vi "AR-Check-Gating.vi"(8 "error in":errorcluster, 10 "Zaber parameters":T3={"Device (dev axis)"="1 3", "Lockstep Group (1)"=1, "Units"=enum."millimeters", "Microstep Size"=4.21875, "Move (units)"=1500.0, "Direction(-1,1)"=0, "Speed (units/s)"=0.0}, 11 "Com ports":T2={"Zaber Com"="COM21", "MCU Com"="COM22", "Laser IP"=""}) -> (0 "error out":errorcluster, 1 "Timed Out":bool=TRUE, 2 "Time Delta (mS)":dbl, 3 "X Pos Triggered":dbl=1500.0)   [LabVIEW 2021]
uses:
  Automation/Zaber Stage/Controls/Zaber-parameters.ctl
  Controls/AR-Interlock-Data.ctl
  Controls/AR-Interlock-monitor-comands.ctl
  Controls/AR-axis-parameters.ctl
panel:
  out "Raw Output 3":string
  out "Raw Output 2":string
  out "Raw Output":string
  in  "Timeout (s)":u32=5
  out "Intlk Data Array":T1[](array[typedef])=[{"Application"="GI", "Msg#"=31, "uS time"=3584961232, "Gate"=FALSE, "Head"=FALSE, "Head Old"=FALSE, "Chamber Ena"=TRUE, "Profiler Ena"=FALSE, "OPower Ena"=FALSE, "Gate Ena"=TRUE, "Time Delta (mS)"=0.0, "Head F Edge"=FALSE}, {"Application"="GI", "Msg#"=32, "uS time"=3633481693, "Gate"=FALSE, "Head"=FALSE, "Head Old"=FALSE, "Chamber Ena"=TRUE, "Profiler Ena"=FALSE, "OPower Ena"=FALSE, "Gate Ena"=TRUE, "Time Delta (mS)"=48520.461, "Head F Edge"=FALSE}] {"Time Delta (mS)" format="%#_3g"}
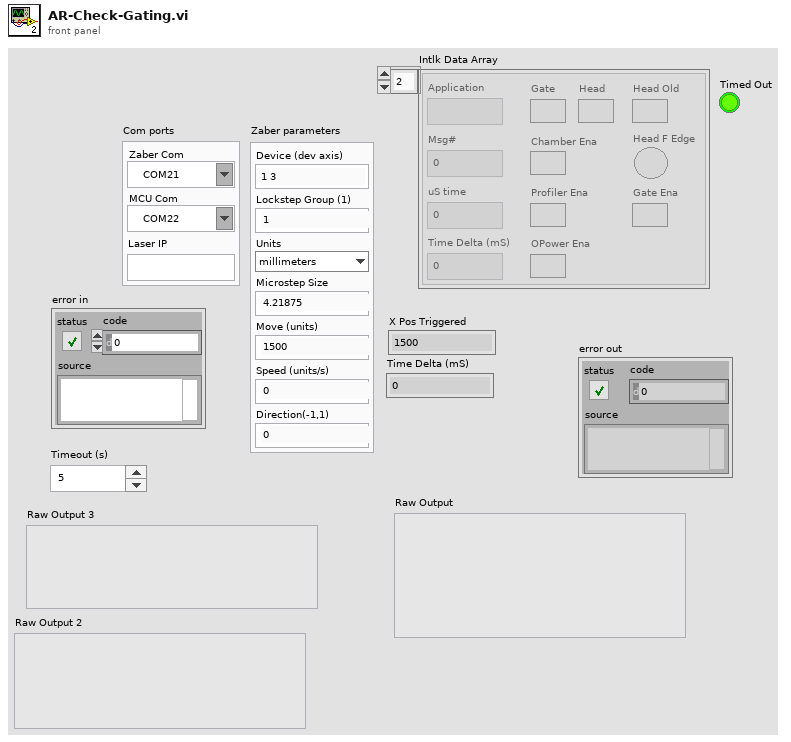
[diagram p1: front panel]
types:
  T1 = typedef "AR-Interlock-Data.ctl" = cluster{"Application":string, "Msg#":i32, "uS time":u32, "Gate":bool, "Head":bool, "Head Old":bool, "Chamber Ena":bool, "Profiler Ena":bool, "OPower Ena":bool, "Gate Ena":bool, "Time Delta (mS)":dbl, "Head F Edge":bool}
  T2 = cluster{"Zaber Com":refnum<visa-resource-name>, "MCU Com":refnum<visa-resource-name>, "Laser IP":string}
  T3 = typedef "Zaber-parameters.ctl" = cluster{"Device (dev axis)":string, "Lockstep Group (1)":u8, "Units":enum16{"microsteps", "microns", "millimeters", "inches", "degrees"}, "Microstep Size":dbl, "Move (units)":dbl, "Direction(-1,1)":i32, "Speed (units/s)":dbl}
  T4 = typedef "AR-Interlock-monitor-comands.ctl" = enum16{"Init", "Request", "Poll Serial", "Close", "Clear Data"}
  T5 = typedef "AR-axis-parameters.ctl" = cluster{"X":T3, "Y":T3}
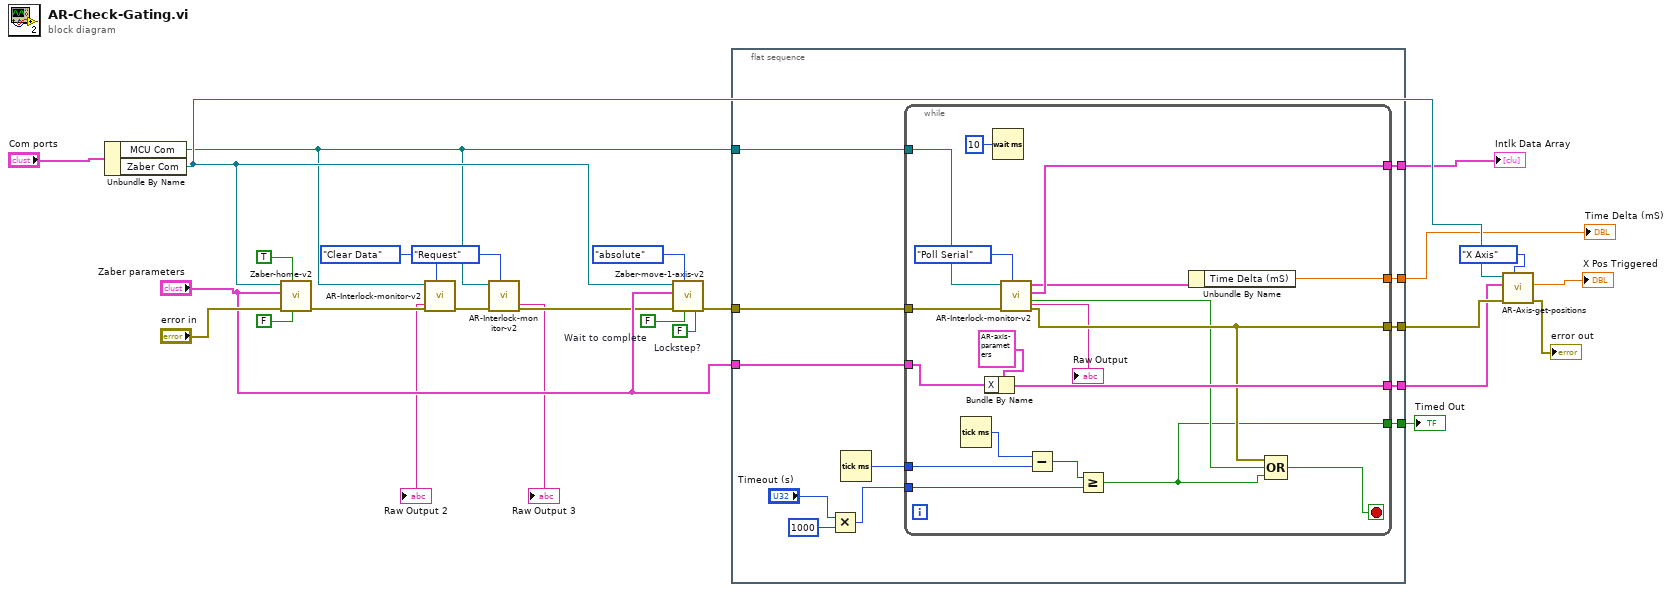
[diagram p0: block diagram]
diagram:
  w25 = FALSE  # Wait to complete
  w24 = FALSE  # Lockstep?
  n1 = Unbundle By Name("Com ports") -> ("MCU Com"=w5:refnum<visa-resource-name>, "Zaber Com"=w16:refnum<visa-resource-name>)
  n2 = call "Zaber-home-v2.vi"("Lockstep?"=FALSE, "Wait to complete"=TRUE, "error in"="error in", "Zaber parameters"="Zaber parameters", "Com Port"=w16) -> ("error out"=w19:errorcluster)  [unwired: 4 in, 2 out]
  n3 = call "AR-Interlock-monitor-v2.vi"("Action"=AR-Interlock-monitor-comands."Clear Data", "error in"=w19, "Inlk Com"=w5) -> ("error out"=w7:errorcluster, "Raw Output"=→"Raw Output 2":string)  [unwired: 4 in, 3 out]
  n4 = call "AR-Interlock-monitor-v2.vi"("Action"=AR-Interlock-monitor-comands."Request", "error in"=w7, "Inlk Com"=w5) -> ("error out"=w6:errorcluster, "Raw Output"=→"Raw Output 3":string)  [unwired: 4 in, 3 out]
  n5 = call "Zaber-move-1-axis-v2.vi"("Lockstep?"=w24, "Wait to complete"=w25, "Movement Type"=enum16{"relative", "absolute"}."absolute", "error in"=w6, "Zaber parameters"="Zaber parameters", "Port In"=w16) -> ("error out"=w17:errorcluster)  [unwired: 3 in, 2 out]
  n6 = flat-sequence {
    tunnel: w17 -> [w38]
    tunnel: w5 -> [w37]
    tunnel: "Zaber parameters" -> [w36]
    tunnel: [w35] -> w14
    tunnel: [w34] -> w13
    tunnel: [w33] -> w11
    tunnel: [w28] -> w10
    tunnel: [w27] -> w3
    frame #0 {
      n7 = Multiply(x="Timeout (s)", y=u32 1000) -> (x*y=w29:u32)
      n8 = Tick Count (ms)() -> (millisecond timer value=w32:u32)
      n9 = while {
        tunnel: w38 -> [w57]
        tunnel: w37 -> [w56]
        tunnel: [w54] -> w33
        tunnel: w36 -> [w52]
        tunnel: [w46] -> w35
        tunnel: [w51] -> w34
        tunnel: w32 -> [w49]
        tunnel: w29 -> [w47]
        tunnel: [w43] -> w28
        tunnel: [w39] -> w27
        stop <- w44 stop-if-true
        n10 = Tick Count (ms)() -> (millisecond timer value=w50:u32)
        n11 = Bundle By Name(cluster=T5 {"X"={"Device (dev axis)"="1 3", "Lockstep Group (1)"=1, "Units"=enum."millimeters", "Microstep Size"=4.21875, "Move (units)"=0.0, "Direction(-1,1)"=1, "Speed (units/s)"=1500.0}, "Y"={"Device (dev axis)"="1", "Lockstep Group (1)"=1, "Units"=enum."millimeters", "Microstep Size"=0.496094, "Move (units)"=0.0, "Direction(-1,1)"=1, "Speed (units/s)"=45.0}} ("Axis params"), "X"=w52) -> (w51:T5)
        n12 = Wait (ms)(milliseconds to wait=u32 10) -> ()  [unwired: 1 out]
        n13 = call "AR-Interlock-monitor-v2.vi"("Action"=AR-Interlock-monitor-comands."Poll Serial", "error in"=w57, "Inlk Com"=w56) -> ("error out"=w46:errorcluster, "Head F Edge"=w45:bool, "Intlk Data Array"=w54:T1[], "Intlk Data"=w40:T1, "Raw Output"=→"Raw Output":string)  [unwired: 4 in]
        n14 = Subtract(x=w50, y=w49) -> (x-y=w48:u32)
        n15 = Greater Or Equal?(x=w48, y=w47) -> (x >= y?=w43:bool)
        n16 = Unbundle By Name(w40) -> ("Time Delta (mS)"=w39:dbl)
        n17 = Compound Arithmetic op=OR(w46, w45, w43) -> (w44:bool)
      }
    }
  }
  n18 = call "AR-Axis-get-positions.vi"("Select"=enum16{"X Axis", "Y Axis", "Both"}."X Axis", "error in"=w14, "Axis params"=w13, "Port In"=w16) -> ("error out"=→"error out":errorcluster, "X Pos"=→"X Pos Triggered":dbl)  [unwired: 4 in, 2 out]
  "Intlk Data Array" <- w11
  "Timed Out" <- w10
  "Time Delta (mS)" <- w3
